vi "CameraRelease.vi"(8 "error in":errorcluster, 11 "Index":i32) -> (0 "error out":errorcluster, 4 "return":i32)   [LabVIEW 2019]
uses:
  [Global] CameraSessionArray.vi
  <vilib>/vision/driver/NI_Vision_Acquisition_Software.lvlib
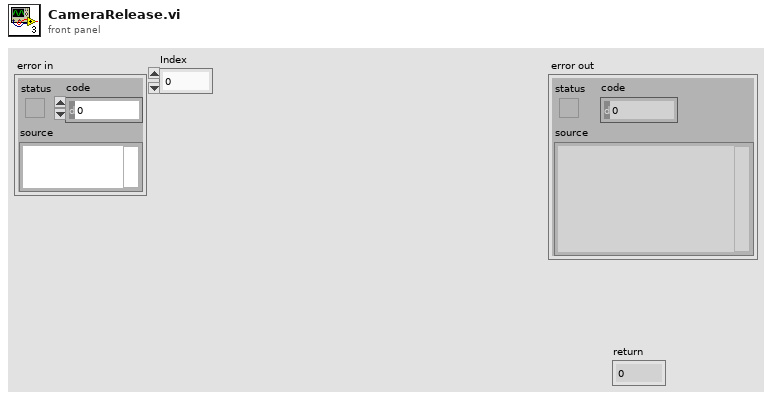
[diagram p1: front panel]
types:
  T1 = typedef "IMAQdx.ctl" = refnum<k21>
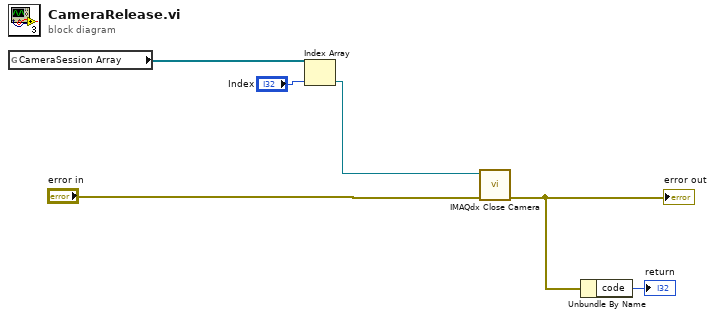
[diagram p0: block diagram]
diagram:
  n1 = global read "[Global] CameraSessionArray.vi" "CameraSession Array"() -> (w3:T1[])
  n2 = Index Array(array=w3, index="Index") -> (element=w1:T1)
  n3 = call <vilib>:"IMAQdx Close Camera.vi"("error in"="error in", "Session In"=w1) -> ("error out"=w5:errorcluster)  [unwired: 9 out]
  "error out" <- w5
  n4 = Unbundle By Name(w5) -> ("code"=→"return":i32)
